vi "Plug_in_Coreolis_lag.vi"() -> (5 "Plug in titles":string[](array[string]), 7 "Plug in values":string[](array[string]))   [LabVIEW 2010]
uses:
  Globals/Plug_in_data_global.vi
  Globals/Meas_global.vi
  <vilib>/Analysis/3filter.llb/Butterworth Filter (DBL).vi
  <vilib>/Analysis/NI_AALPro.lvlib
  <vilib>/Analysis/NI_AALBase.lvlib
panel:
  in  "filter type":T1(ring)
  in  "fh":dbl=140.0 format="%.2f"
  out "Standard Deviation":dbl(graph)
  in  "order":i32=3
  out "mean":dbl format="%^.3e"
  out "Lag (s)":dbl(graph)
  in  "fl":dbl=150.0 format="%.2f"
  out "df":dbl format="%.2f"
  out "peak freq.":dbl format="%.2f"
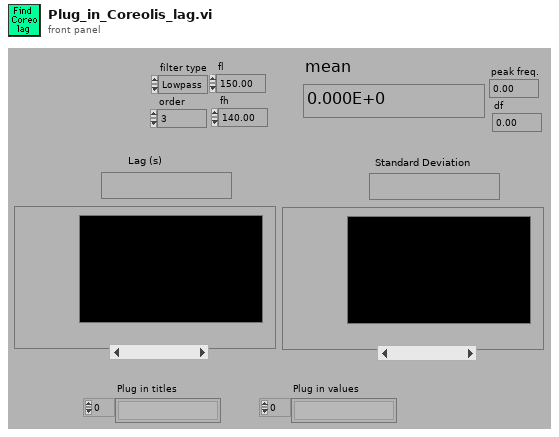
[diagram p1: front panel]
types:
  T1 = enum32{"Lowpass", "Highpass", "Bandpass", "Bandstop"}
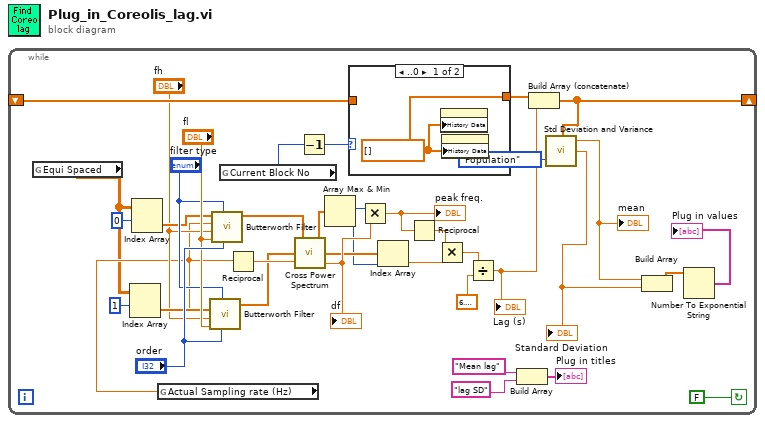
[diagram p0: block diagram]
diagram:
  n1 = while {
    shift-left: _ -> [w17]
    shift-right: [w15] -> _
    stop <- FALSE continue-if-true
    n2 = global read "Plug_in_data_global.vi" "Equi Spaced"() -> (w8:dbl[][])
    n3 = Index Array(array=w8, index (row)=1) -> (element=w27:dbl[])  [unwired: 1 in]
    n4 = Index Array(array=w8, index (row)=0) -> (element=w25:dbl[])  [unwired: 1 in]
    n5 = global read "Meas_global.vi" "Actual Sampling rate (Hz)"() -> (w9:dbl)
    n6 = call-poly <vilib>:"Butterworth Filter.vi"("order"="order", "filter type"="filter type", "low cutoff freq: fl"="fl", "high cutoff freq: fh"="fh", "sampling freq: fs"=w9, "X"=w27) -> ("Filtered X"=w31:dbl[])  [unwired: 2 in, 1 out]
    n7 = call-poly <vilib>:"Butterworth Filter.vi"("order"="order", "filter type"="filter type", "low cutoff freq: fl"="fl", "high cutoff freq: fh"="fh", "sampling freq: fs"=w9, "X"=w25) -> ("Filtered X"=w30:dbl[])  [unwired: 2 in, 1 out]
    n8 = global read "Meas_global.vi" "Current Block No"() -> (w10:i32)
    n9 = Reciprocal(x=w9) -> (1/x=w34:dbl)
    n10 = call <vilib>:"Cross Power Spectrum.vi"("dt"=w34, "Signal Y (V)"=w31, "Signal X (V)"=w30) -> ("df"=w24:dbl, "Cross Power XY Spectrum Phase (radians)"=w23:dbl[], "Cross Power XY Spectrum Mag (V^2rms)"=w22:dbl[])
    "df" <- w24
    n11 = Decrement(x=w10) -> (x-1=w14:i32)
    n12 = Array Max & Min(array=w22) -> (max index (indices)=w21:i32)  [unwired: 3 out]
    n13 = case shown="..0" w14 {
      tunnel: w17 -> [_ w39]
      tunnel: [w38 w39] -> w16
      frame ..0 {
        w38 = dbl[] [] ("History Data")
        n14 = property on="Standard Deviation" class="WFChart (strict)"("History Data"=w38) -> ()  [unwired: 2 in, 2 out]
        n15 = property on="Lag (s)" class="WFChart (strict)"("History Data"=w38) -> ()  [unwired: 2 in, 2 out]
      }
      frame 1.. {
      }
    }
    n16 = Multiply(x=w21, y=w24) -> (x*y=w36:dbl)
    "peak freq." <- w36
    n17 = Index Array(array=w23, index=w21) -> (element=w35:dbl)
    n18 = Reciprocal(x=w36) -> (1/x=w37:dbl)
    n19 = Multiply(x=w37, y=w35) -> (x*y=w32:dbl)
    n20 = Divide(x=w32, y=6.283185307179586) -> (x/y=w18:dbl)
    "Lag (s)" <- w18
    n21 = Build Array("Mean lag", "lag SD") -> (→"Plug in titles":string[])
    n22 = Build Array (concatenate)(w16, w18) -> (w15:dbl[])
    n23 = call <vilib>:"Std Deviation and Variance.vi"("X"=w15, "Weighting (Sample)"=enum16{"Sample", "Population"}."Population") -> ("mean"=w6:dbl, "standard deviation"=w5:dbl)  [unwired: 1 out]
    "mean" <- w6
    "Standard Deviation" <- w5
    n24 = Build Array(w6, w5) -> (w4:dbl[])
    n25 = Number To Exponential String(number=w4) -> (E-format string=→"Plug in values":string[])  [unwired: 3 in]
  }
